vi "set gain.vi"(8 "error in (no error)":errorcluster, 11 "Thorcam in":refnum<class "Thorcam.lvclass">) -> (0 "error out":errorcluster, 3 "Thorcam out":refnum<class "Thorcam.lvclass">)   [LabVIEW 2012, in "Thorcam.lvclass"]
uses:
  Thorcam.lvclass
  Thorcam.lvclass/Thorcam.ctl
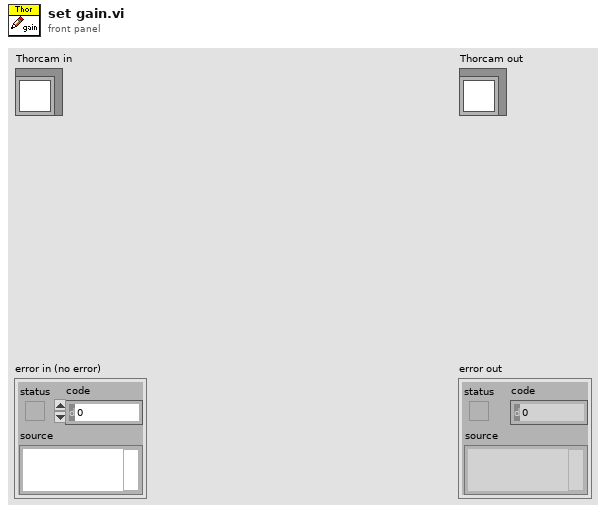
[diagram p1: front panel]
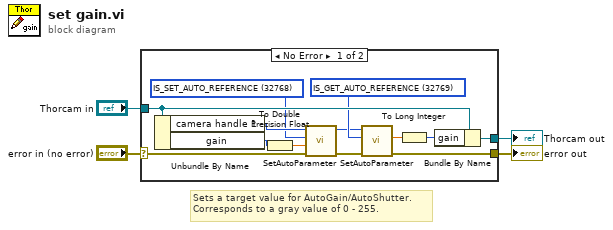
[diagram p0: block diagram]
diagram:
  # "Sets a target value for AutoGain/AutoShutter.\nCorresponds to a gray value of 0 - 255."
  n1 = case shown="No Error" "error in (no error)" {
    selector: "error in (no error)" -> [w15 w19]
    tunnel: [w7 w19] -> w3
    tunnel: [w16 w18] -> w1
    tunnel: "Thorcam in" -> [w17 w18]
    frame No Error {
      w9 = 32769 items=["IS_SET_ENABLE_AUTO_GAIN"=34816, "IS_GET_ENABLE_AUTO_GAIN"=34817, "IS_SET_ENABLE_AUTO_SHUTTER"=34818, "IS_GET_ENABLE_AUTO_SHUTTER"=34819, "IS_SET_ENABLE_AUTO_WHITEBALANCE"=34820, "IS_GET_ENABLE_AUTO_WHITEBALANCE"=34821, "IS_SET_ENABLE_AUTO_FRAMERATE"=34822, "IS_GET_ENABLE_AUTO_FRAMERATE"=34823, "IS_SET_AUTO_REFERENCE"=32768, "IS_GET_AUTO_REFERENCE"=32769, "IS_SET_AUTO_GAIN_MAX"=32770, "IS_GET_AUTO_GAIN_MAX"=32771, "IS_SET_AUTO_SHUTTER_MAX"=32772, "IS_GET_AUTO_SHUTTER_MAX"=32773, "IS_SET_AUTO_SPEED"=32774, "IS_GET_AUTO_SPEED"=32775, "IS_SET_AUTO_WB_OFFSET"=32776, "IS_GET_AUTO_WB_OFFSET"=32777, "IS_SET_AUTO_WB_GAIN_RANGE"=32778, "IS_GET_AUTO_WB_GAIN_RANGE"=32779, "IS_SET_AUTO_WB_SPEED"=32780, "IS_GET_SUTO_WB_SPEED"=32781, "IS_SET_AUTO_WB_ONCE"=32782, "IS_GET_AUTO_WB_ONCE"=32783] ("Param")
      w13 = 32768 items=["IS_SET_ENABLE_AUTO_GAIN"=34816, "IS_GET_ENABLE_AUTO_GAIN"=34817, "IS_SET_ENABLE_AUTO_SHUTTER"=34818, "IS_GET_ENABLE_AUTO_SHUTTER"=34819, "IS_SET_ENABLE_AUTO_WHITEBALANCE"=34820, "IS_GET_ENABLE_AUTO_WHITEBALANCE"=34821, "IS_SET_ENABLE_AUTO_FRAMERATE"=34822, "IS_GET_ENABLE_AUTO_FRAMERATE"=34823, "IS_SET_AUTO_REFERENCE"=32768, "IS_GET_AUTO_REFERENCE"=32769, "IS_SET_AUTO_GAIN_MAX"=32770, "IS_GET_AUTO_GAIN_MAX"=32771, "IS_SET_AUTO_SHUTTER_MAX"=32772, "IS_GET_AUTO_SHUTTER_MAX"=32773, "IS_SET_AUTO_SPEED"=32774, "IS_GET_AUTO_SPEED"=32775, "IS_SET_AUTO_WB_OFFSET"=32776, "IS_GET_AUTO_WB_OFFSET"=32777, "IS_SET_AUTO_WB_GAIN_RANGE"=32778, "IS_GET_AUTO_WB_GAIN_RANGE"=32779, "IS_SET_AUTO_WB_SPEED"=32780, "IS_GET_SUTO_WB_SPEED"=32781, "IS_SET_AUTO_WB_ONCE"=32782, "IS_GET_AUTO_WB_ONCE"=32783] ("Param")
      n2 = Unbundle By Name(w17) -> ("camera handle 1"=w14:u32, "gain"=w12:i32)
      n3 = To Double Precision Float(number=w12) -> (double precision float=w11:dbl)
      n4 = call <instrlib>:"SetAutoParameter.vi"("error in"=w15, "Set Value"=w11, "Param"=w13, "Camera Handle In"=w14) -> ("error out"=w10:errorcluster, "Camera Handle Out"=w8:u32)  [unwired: 5 in, 1 out]
      n5 = call <instrlib>:"SetAutoParameter.vi"("error in"=w10, "Param"=w9, "Camera Handle In"=w8) -> ("error out"=w7:errorcluster, "Value"=w5:dbl)  [unwired: 6 in, 1 out]
      n6 = To Long Integer(number=w5) -> (32bit integer=w6:i32)
      n7 = Bundle By Name(cluster=w17, "gain"=w6) -> (w16:refnum<class "Thorcam.lvclass">)
    }
    frame Error {
    }
  }
  "error out" <- w3
  "Thorcam out" <- w1
